vi "FTW-CodeGen-AdaptToInputs.vi"(0 "State In":T1, 5 "XRef":refnum<vi>, 7 "Term Types":cluster{"Type":variant, "ID":string}[](array[cluster])) -> (4 "State Out":T1, 6 "Reply":string[](array[string]))   [LabVIEW 2015, in "FTW-Dataflow-Synchronizer.xnode"]
uses:
  FTW-Dataflow-Synchronizer.xnode
  FTW-CodeGen-State.ctl
  FTW-CodeGen-XNodeReplyType.ctl
panel:
  # "Inputs"
  # "Outputs"
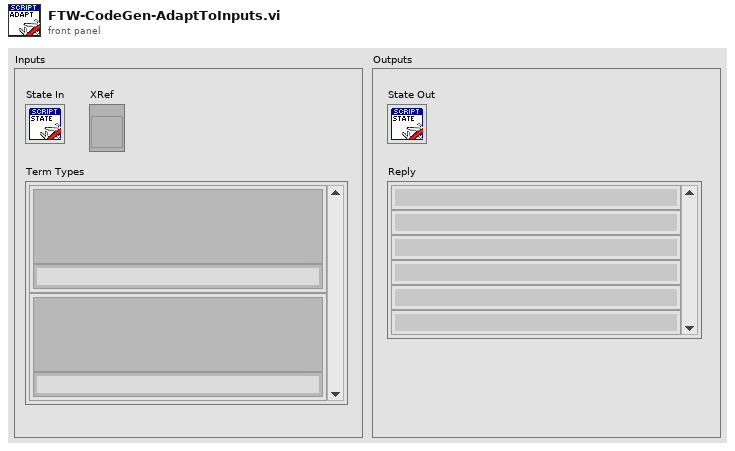
[diagram p1: front panel]
types:
  T1 = typedef "FTW-Dataflow-Synchronizer.xnode/FTW-CodeGen-State.ctl" = cluster{"InputTerminals":cluster{"Wired?":bool, "ID":string, "DataName":string, "DataColor":u32, "Type":variant}[], "EnableTiming?":bool}
  T2 = typedef "FTW-CodeGen-XNodeReplyType.ctl" = enum16{"UpdateState", "AdaptToInputs", "AdaptAndAugment", "CosmeticUpdate", "NoReply"}
  T3 = cluster{"Wired?":bool, "ID":string, "DataName":string, "DataColor":u32, "Type":variant}[]
  T4 = cluster{"Wired?":bool, "ID":string, "DataName":string, "DataColor":u32, "Type":variant}
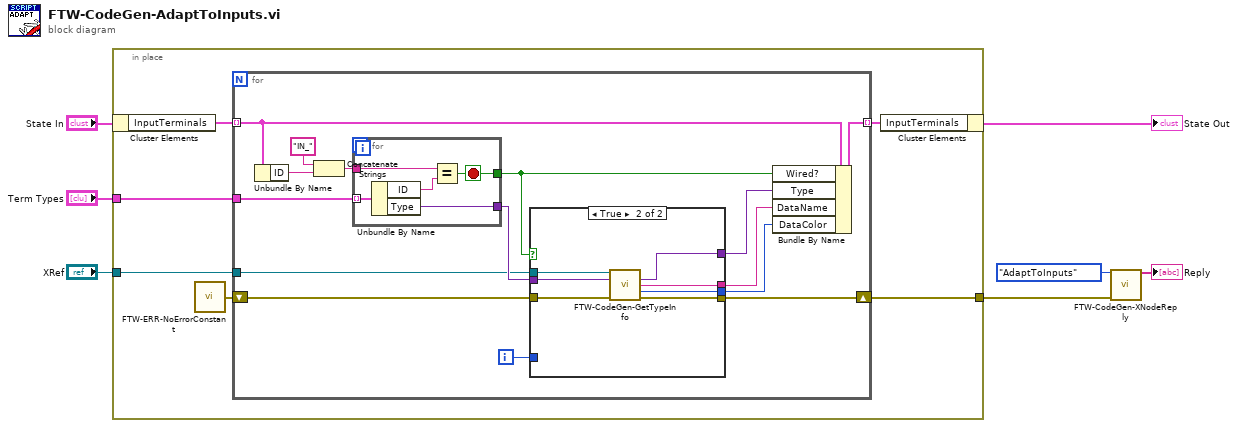
[diagram p0: block diagram]
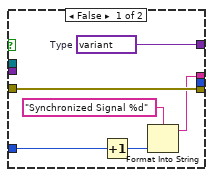
[diagram p2: hidden frame]
diagram:
  n1 = in-place {
    in-place-border: "Term Types" -> [w9]
    in-place-border: [w12] -> w5
    in-place-border: "XRef" -> [w8]
    n2 = in-place-cluster #1("State In") -> ("InputTerminals"=w11:T3)
    n3 = call "FTW-ERR-NoErrorConstant.vi"() -> ("no error"=w13:errorcluster)
    n4 = for {
      shift-right: [w28] -> w12
      shift-left: w13 -> [w20]
      tunnel: w11 -> [w26] mode=indexing
      tunnel: [w27] -> w10 mode=indexing
      tunnel: w9 -> [w23]
      tunnel: w8 -> [w19]
      i -> [w14]
      n5 = Unbundle By Name(w26) -> ("ID"=w24:string)
      n6 = Concatenate Strings("IN_" ("format string"), w24) -> (w22:string)
      n7 = for {
        tunnel: [w46] -> w21
        tunnel: [w45] -> w15
        tunnel: w23 -> [w44] mode=indexing
        tunnel: w22 -> [w42]
        stop <- w45 stop-if-true
        n8 = Unbundle By Name(w44) -> ("ID"=w43:string, "Type"=w46:variant)
        n9 = Equal?(x=w42, y=w43) -> (x = y?=w45:bool)
      }
      n10 = case shown="True" w15 {
        tunnel: [w34 w41] -> w28
        tunnel: w21 -> [_ w40]
        tunnel: w20 -> [w34 w39]
        tunnel: w19 -> [_ w38]
        tunnel: [w29 w37] -> w18
        tunnel: [_ w36] -> w17
        tunnel: [w33 w35] -> w16
        tunnel: w14 -> [w30 _]
        frame False {
          w33 = variant(variant variant)  # Type
          n11 = Increment(x=w30) -> (x+1=w32:i32)
          n12 = Format Into String(format string="Synchronized Signal %d" ("Name"), w32) -> (resulting string=w29:string)  [unwired: 2 in, 1 out]
        }
        frame True {
          n13 = call "FTW-CodeGen-GetTypeInfo.vi"("XRef"=w38, "Type Information In"=w40, "error in"=w39) -> ("Safe Type Information for this Context"=w35:variant, "Data Name"=w37:string, "Data Type Color"=w36:u32, "error out"=w41:errorcluster)  [unwired: 9 in]
        }
      }
      n14 = Bundle By Name(cluster=w26, "Wired?"=w15, "Type"=w16, "DataName"=w18, "DataColor"=w17) -> (w27:T4)
    }
    n15 = in-place-cluster #1("InputTerminals"=w10) -> (→"State Out":T1)
  }
  n16 = call "FTW-CodeGen-XNodeReply.vi"("XNode Reply Type"=FTW-CodeGen-XNodeReplyType."AdaptToInputs", "error in"=w5) -> ("Reply"=→"Reply":string[])  [unwired: 13 in]
